vi "Add Regex Scrubber.vi"   [LabVIEW 2020, in "Approval Tests.lvlib"]
doc: "Drops everything needed to scrub using a regex with a static replacement."
uses:
  Approval Tests.lvlib
  Options/Options.lvclass
  Regex Scrubber/Regex Scrubber.lvclass
  C:/Users/SAS/Desktop/ApprovalTests.LabVIEW/Source/Approval Tests/Scrubber/Scrubber.lvclass
  Regex Scrubber/Regex Scrubber.lvclass/Regex Scrubber.ctl
  Regex Scrubber/Write Regex.vi
  Regex Scrubber/Write Replacement.vi
  Options/Write Add Scrubber.vi
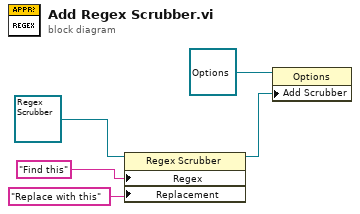
[diagram p0: block diagram]
diagram:
  n1 = property class="Regex Scrubber"(reference=refnum<class "Regex Scrubber.lvclass"> refnum ("Approval Tests.lvlib:Regex Scrubber"), "Regex"="Find this", "Replacement"="Replace with this") -> (reference out=w1:refnum<class "Regex Scrubber.lvclass">)  [unwired: 1 in, 1 out]
  n2 = property class="Options"(reference=refnum<class "Options.lvclass"> refnum ("Approval Tests.lvlib:Options"), "Add Scrubber"=w1) -> ()  [unwired: 1 in, 2 out]
